vi "_CallQueue.vi"() -> ()   [LabVIEW 2019]
panel:
  in  "stop":bool
  out "Valid?":bool
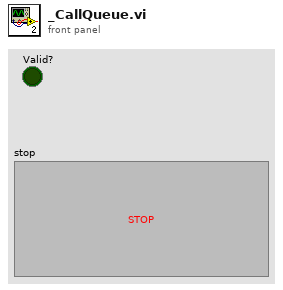
[diagram p1: front panel]
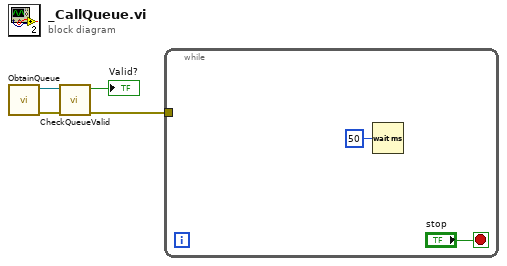
[diagram p0: block diagram]
diagram:
  n1 = call "ObtainQueue.vi"() -> ("error out"=w3:errorcluster, "queue out"=w4:refnum<queue>)  [unwired: 10 in]
  n2 = call "CheckQueueValid.vi"("error in (no error)"=w3, "queue out"=w4) -> ("error out"=w1:errorcluster, "Valid?"=→"Valid?":bool)  [unwired: 8 in]
  n3 = while {
    tunnel: w1 -> [_]
    stop <- "stop" stop-if-true
    n4 = Wait (ms)(milliseconds to wait=u32 50) -> ()  [unwired: 1 out]
  }
